vi "Get VISA Session.vi"(8 "error in":errorcluster, 11 "Scope VISA in":refnum<class "Scope VISA.lvclass">) -> (0 "error out":errorcluster, 2 "VISA session":refnum<visa-resource-name>, 3 "Scope VISA out":refnum<class "Scope VISA.lvclass">)   [LabVIEW 2023, in "Scope VISA.lvlib" / "Scope VISA.lvclass"]
uses:
  Scope VISA.lvclass
  Scope VISA.lvclass/Scope VISA.ctl
  Scope Base/Scope Base.lvclass
  Configuration/Scope VISA CFG.lvclass
  D:/git/HAL/Scope Base/Scope Base.lvclass
  D:/git/HAL/Hardware_class/Instrument.lvclass
  D:/git/HAL/Interfaces/IScope/IScope.lvclass
  D:/git/HAL/Scope VISA/Scope VISA.lvclass
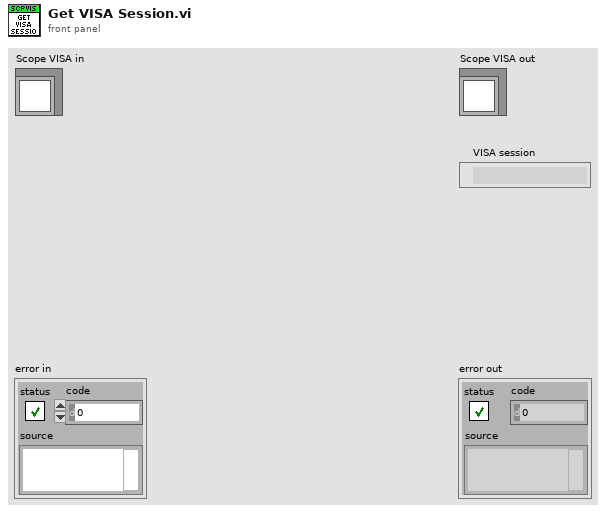
[diagram p1: front panel]
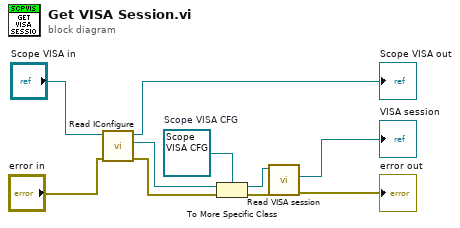
[diagram p0: block diagram]
diagram:
  w6 = refnum<class "Scope VISA CFG.lvclass"> refnum  # Scope VISA CFG
  n1 = call "Read IConfigure.vi"("error in (no error)"="error in", "Scope Base in"="Scope VISA in") -> ("error out"=w8:errorcluster, "IConfigure"=w7:refnum<class "IConfigure.lvclass">, "Scope Base out"=→"Scope VISA out":refnum<class "Scope VISA.lvclass">)  [unwired: 7 in]
  n2 = To More Specific Class(target class=w6, reference=w7, error in=w8) -> (specific class reference=w3:refnum<class "Scope VISA CFG.lvclass">, error out=w5:errorcluster)
  n3 = call "Read VISA session.vi"("error in (no error)"=w5, "Scope VISA CFG in"=w3) -> ("error out"=→"error out":errorcluster, "VISA session"=→"VISA session":refnum<visa-resource-name>)  [unwired: 7 in, 1 out]
